vi "Add FIFO Publisher Command.vi"(8 "error in":errorcluster, 10 "New FIFO Pub":T1, 11 "ChanMngOOB_Rx in":refnum<class "ChanMngOOB_Rx.lvclass">) -> (0 "error out":errorcluster, 3 "ChanMngOOB_Rx out":refnum<class "ChanMngOOB_Rx.lvclass">)   [LabVIEW 2021, in "ChanMngOOB_Rx.lvclass"]
uses:
  ChanMngOOB_Rx.lvclass
  C:/Program Files/National Instruments/LabVIEW 2021/vi.lib/CIF Foundation/CIF Out of Band Commands/CIFOutOfBand.lvclass
  Typedef/FIFO Publisher.ctl
  <vilib>/CIF Foundation/CIF Channels Core/ChannelCommon/typedef/New FIFO Instance Configuration.ctl
  <vilib>/CIF Foundation/CIF Out of Band Commands/CIFOutOfBand.lvclass/CIFOutOfBand.ctl
  <vilib>/CIF Foundation/CIF Out of Band Commands/Typedef/OOB Container.ctl
  Typedef/OOB ChnMng Commands.ctl
  Typedef/Template Payload.ctl
  Typedef/Channel Connection Data.ctl
  Typedef/Channel Fault Data.ctl
  <vilib>/CIF Foundation/CIF Out of Band Commands/CIFOutOfBand.lvclass
  <vilib>/CIF Foundation/CIF Channels Core/ChannelCommon/ChannelCommon.lvlib
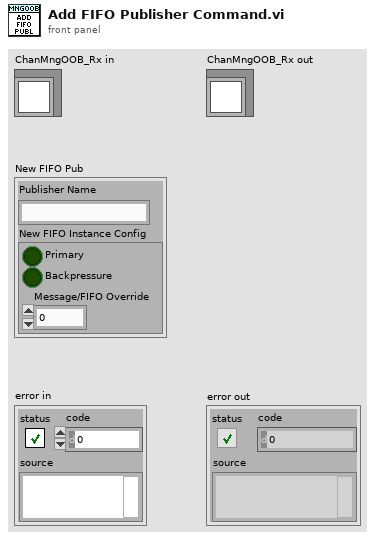
[diagram p1: front panel]
types:
  T1 = typedef "ChanMngOOB_Rx.lvclass/FIFO Publisher.ctl" = cluster{"Publisher Name":string, "New FIFO Instance Config":T2}
  T2 = typedef "ChannelCommon.lvlib/New FIFO Instance Configuration.ctl" = cluster{"Primary":bool, "Backpressure":bool, "Message/FIFO Override":u32}
  T3 = typedef "CIFOutOfBand.lvclass/OOB Container.ctl" = cluster{"Commands (bitwise)":u64, "Payload":variant}
  T4 = typedef "ChanMngOOB_Rx.lvclass/OOB ChnMng Commands.ctl" = enum8{"Connect Channel", "Force Channel", "Add FIFO Pub", "Remove FIFO Pub"}
  T5 = typedef "ChanMngOOB_Rx.lvclass/Template Payload.ctl" = cluster{"Connections":T6[], "Forces":T7[], "FIFO Pub":T1}
  T6 = typedef "ChanMngOOB_Rx.lvclass/Channel Connection Data.ctl" = cluster{"Publisher Name":string, "Subscriber Name":string, "Connection Data":u8[]}
  T7 = typedef "ChanMngOOB_Rx.lvclass/Channel Fault Data.ctl" = cluster{"Channel Name":string, "Force Data":u8[], "Force Active":bool}
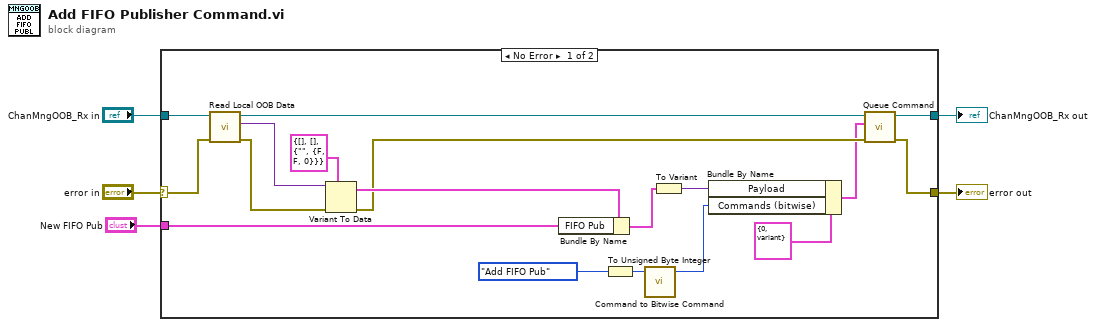
[diagram p0: block diagram]
diagram:
  n1 = case shown="No Error" "error in" {
    selector: "error in" -> [w20 w25]
    tunnel: [w22 w25] -> w4
    tunnel: "ChanMngOOB_Rx in" -> [w21 w24]
    tunnel: [w23 w24] -> w2
    tunnel: "New FIFO Pub" -> [w6 _]
    frame No Error {
      n2 = call <vilib>:"Read Local OOB Data.vi"("error in"=w20, "OOB in"=w21) -> ("error out"=w16:errorcluster, "Local OOB Data"=w19:variant, "OOB out"=w9:refnum<class "ChanMngOOB_Rx.lvclass">)  [unwired: 7 in]
      n3 = Variant To Data(error in=w16, type=T5 {"Connections"=[], "Forces"=[], "FIFO Pub"={"Publisher Name"="", "New FIFO Instance Config"={"Primary"=FALSE, "Backpressure"=FALSE, "Message/FIFO Override"=0}}} ("Template Payload"), Variant=w19) -> (data=w17:T5, error out=w10:errorcluster)
      n4 = Bundle By Name(cluster=w17, "FIFO Pub"=w6) -> (w13:T5)
      n5 = To Unsigned Byte Integer(number=OOB_ChnMng_Commands."Add FIFO Pub" ("OOB Main Commands")) -> (unsigned 8bit integer=w15:u8)
      n6 = call <vilib>:"Command to Bitwise Command.vi"("Command"=w15) -> ("bit command"=w8:u64)  [unwired: 3 in]
      n7 = To Variant(anything=w13) -> (Variant=w11:variant)
      n8 = Bundle By Name(cluster=T3 {"Commands (bitwise)"=0, "Payload"=variant} ("OOB Data"), "Payload"=w11, "Commands (bitwise)"=w8) -> (w7:T3)
      n9 = call <vilib>:"Queue Command.vi"("error in"=w10, "OOB Data"=w7, "OOB in"=w9) -> ("error out"=w22:errorcluster, "OOB out"=w23:refnum<class "ChanMngOOB_Rx.lvclass">)  [unwired: 7 in]
    }
    frame Error {
    }
  }
  "error out" <- w4
  "ChanMngOOB_Rx out" <- w2
